vi "Read Calibrations + Settings from Dash 2016.vi"   [LabVIEW 2015]
uses:
  <vilib>/Rock Robotics/Network Tables/NT Read Numeric Array.vi
  Global Variables/Calibrations.vi
  Global Variables/Settings.vi
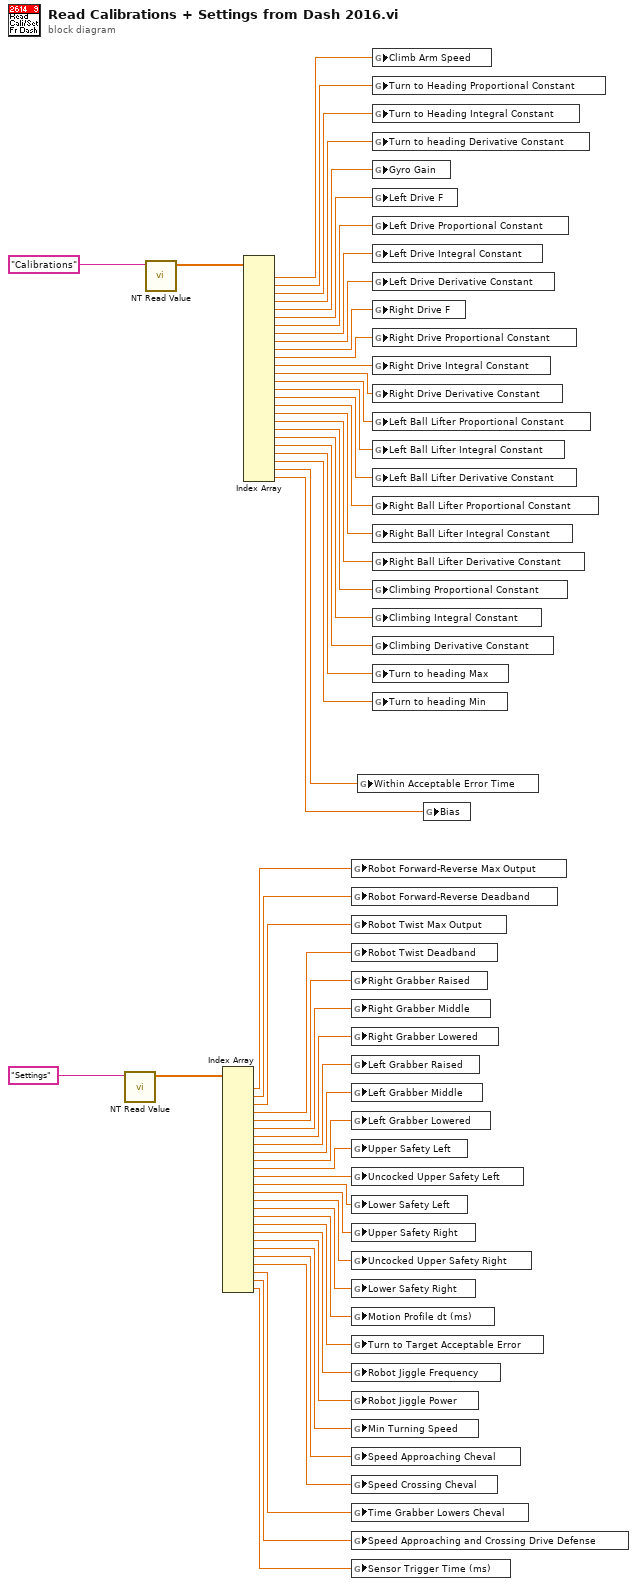
[diagram p0: block diagram]
diagram:
  n1 = call-poly <vilib>:"NT Read Value.vi"("Name"="Settings") -> ("Numeric Array"=w9:dbl[])  [unwired: 9 in, 1 out]
  n2 = call-poly <vilib>:"NT Read Value.vi"("Name"="Calibrations") -> ("Numeric Array"=w30:dbl[])  [unwired: 9 in, 1 out]
  n3 = Index Array(array=w9) -> (element #1=w29:dbl, element #2=w28:dbl, element #3=w21:dbl, element #4=w27:dbl, element #5=w26:dbl, element #6=w25:dbl, element #7=w24:dbl, element #8=w23:dbl, element #9=w22:dbl, element #10=w20:dbl, element #11=w19:dbl, element #12=w18:dbl, element #13=w17:dbl, element #14=w16:dbl, element #15=w15:dbl, element #16=w14:dbl, element #17=w13:dbl, element #18=w12:dbl, element #19=w11:dbl, element #20=w10:dbl, element #21=w8:dbl, element #22=w7:dbl, element #23=w6:dbl, element #24=w5:dbl, element #25=w4:dbl, element #26=w3:dbl)  [unwired: 26 in]
  n4 = Index Array(array=w30) -> (element #1=w33:dbl, element #2=w54:dbl, element #3=w53:dbl, element #4=w37:dbl, element #5=w52:dbl, element #6=w51:dbl, element #7=w49:dbl, element #8=w50:dbl, element #9=w48:dbl, element #10=w47:dbl, element #11=w44:dbl, element #12=w46:dbl, element #13=w45:dbl, element #14=w43:dbl, element #15=w42:dbl, element #16=w41:dbl, element #17=w40:dbl, element #18=w39:dbl, element #19=w38:dbl, element #20=w34:dbl, element #21=w35:dbl, element #22=w36:dbl, element #23=w32:dbl, element #24=w31:dbl, element #25=w2:dbl, element #26=w1:dbl)  [unwired: 26 in]
  n5 = global write "Settings.vi" "Robot Forward-Reverse Max Output"(w29) -> ()
  n6 = global write "Settings.vi" "Robot Forward-Reverse Deadband"(w28) -> ()
  n7 = global write "Settings.vi" "Robot Twist Max Output"(w21) -> ()
  n8 = global write "Settings.vi" "Robot Twist Deadband"(w27) -> ()
  n9 = global write "Settings.vi" "Right Grabber Raised"(w26) -> ()
  n10 = global write "Settings.vi" "Right Grabber Middle"(w25) -> ()
  n11 = global write "Settings.vi" "Right Grabber Lowered"(w24) -> ()
  n12 = global write "Settings.vi" "Left Grabber Raised"(w23) -> ()
  n13 = global write "Settings.vi" "Left Grabber Middle"(w22) -> ()
  n14 = global write "Settings.vi" "Left Grabber Lowered"(w20) -> ()
  n15 = global write "Settings.vi" "Upper Safety Left"(w19) -> ()
  n16 = global write "Settings.vi" "Uncocked Upper Safety Left"(w18) -> ()
  n17 = global write "Settings.vi" "Lower Safety Left"(w17) -> ()
  n18 = global write "Settings.vi" "Upper Safety Right"(w16) -> ()
  n19 = global write "Settings.vi" "Uncocked Upper Safety Right"(w15) -> ()
  n20 = global write "Settings.vi" "Lower Safety Right"(w14) -> ()
  n21 = global write "Settings.vi" "Motion Profile dt (ms)"(w13) -> ()
  n22 = global write "Settings.vi" "Turn to Target Acceptable Error"(w12) -> ()
  n23 = global write "Settings.vi" "Robot Jiggle Frequency"(w11) -> ()
  n24 = global write "Settings.vi" "Robot Jiggle Power"(w10) -> ()
  n25 = global write "Settings.vi" "Min Turning Speed"(w8) -> ()
  n26 = global write "Settings.vi" "Speed Approaching Cheval"(w7) -> ()
  n27 = global write "Settings.vi" "Speed Crossing Cheval"(w6) -> ()
  n28 = global write "Settings.vi" "Time Grabber Lowers Cheval"(w5) -> ()
  n29 = global write "Settings.vi" "Speed Approaching and Crossing Drive Defense"(w4) -> ()
  n30 = global write "Settings.vi" "Sensor Trigger Time (ms)"(w3) -> ()
  n31 = global write "Calibrations.vi" "Within Acceptable Error Time"(w2) -> ()
  n32 = global write "Calibrations.vi" "Climb Arm Speed"(w33) -> ()
  n33 = global write "Calibrations.vi" "Turn to Heading Proportional Constant"(w54) -> ()
  n34 = global write "Calibrations.vi" "Turn to Heading Integral Constant"(w53) -> ()
  n35 = global write "Calibrations.vi" "Turn to heading Derivative Constant"(w37) -> ()
  n36 = global write "Calibrations.vi" "Gyro Gain"(w52) -> ()
  n37 = global write "Calibrations.vi" "Left Drive F"(w51) -> ()
  n38 = global write "Calibrations.vi" "Left Drive Proportional Constant"(w49) -> ()
  n39 = global write "Calibrations.vi" "Left Drive Integral Constant"(w50) -> ()
  n40 = global write "Calibrations.vi" "Left Drive Derivative Constant"(w48) -> ()
  n41 = global write "Calibrations.vi" "Right Drive F"(w47) -> ()
  n42 = global write "Calibrations.vi" "Right Drive Proportional Constant"(w44) -> ()
  n43 = global write "Calibrations.vi" "Right Drive Integral Constant"(w46) -> ()
  n44 = global write "Calibrations.vi" "Right Drive Derivative Constant"(w45) -> ()
  n45 = global write "Calibrations.vi" "Left Ball Lifter Proportional Constant"(w43) -> ()
  n46 = global write "Calibrations.vi" "Left Ball Lifter Integral Constant"(w42) -> ()
  n47 = global write "Calibrations.vi" "Left Ball Lifter Derivative Constant"(w41) -> ()
  n48 = global write "Calibrations.vi" "Right Ball Lifter Proportional Constant"(w40) -> ()
  n49 = global write "Calibrations.vi" "Right Ball Lifter Integral Constant"(w39) -> ()
  n50 = global write "Calibrations.vi" "Right Ball Lifter Derivative Constant"(w38) -> ()
  n51 = global write "Calibrations.vi" "Climbing Proportional Constant"(w34) -> ()
  n52 = global write "Calibrations.vi" "Climbing Integral Constant"(w35) -> ()
  n53 = global write "Calibrations.vi" "Climbing Derivative Constant"(w36) -> ()
  n54 = global write "Calibrations.vi" "Turn to heading Max"(w32) -> ()
  n55 = global write "Calibrations.vi" "Turn to heading Min"(w31) -> ()
  n56 = global write "Calibrations.vi" "Bias"(w1) -> ()
